vi "TIO Stream Read_Ser.vi"(8 "error in (no error)":errorcluster, 11 "VISA resource name":refnum<visa-resource-name>) -> (0 "error out":errorcluster, 1 "Payload":string, 2 "Type":T1(ring)=enum."RPC Request", 3 "VISA resource name Out":refnum<visa-resource-name>, 4 "Payload Length":u16)   [LabVIEW 2019]
uses:
  <userlib>/TIO Library 2010/TIO Serial Checksum CRC32.vi
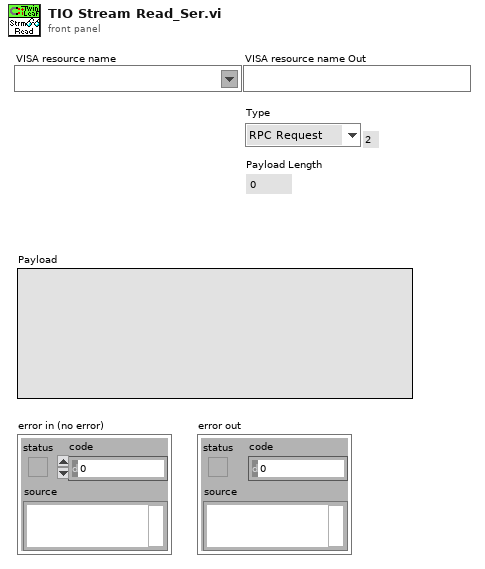
[diagram p1: front panel]
types:
  T1 = enum8{"Invalid", "Log", "RPC Request", "RPC Reply", "RPC Error", "Stream Description", "User"}
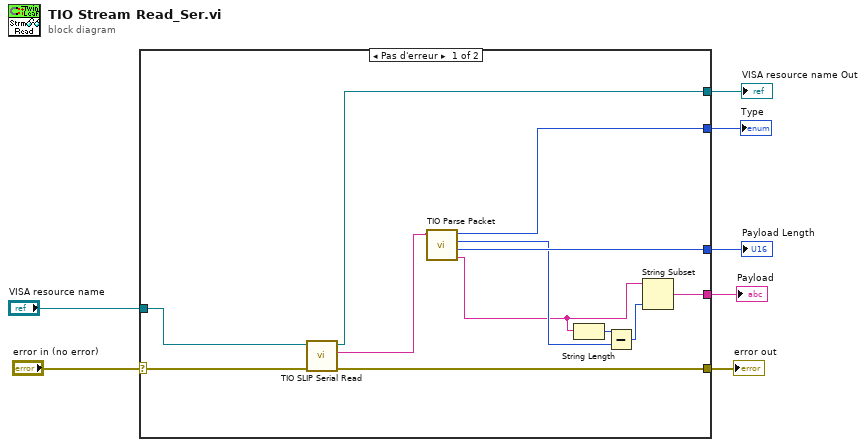
[diagram p0: block diagram]
diagram:
  n1 = case shown="Pas d'erreur" "error in (no error)" {
    selector: "error in (no error)" -> [w9 w20]
    tunnel: [w19 w20] -> w7
    tunnel: [w18 _] -> w6
    tunnel: [w17 _] -> w5
    tunnel: [w12 _] -> w4
    tunnel: "VISA resource name" -> [w10 w21]
    tunnel: [w8 w21] -> w1
    frame No Error {
      n2 = call <userlib>:"TIO SLIP Serial Read.vi"("error in (no error)"=w9, "VISA resource name"=w10) -> ("error out"=w19:errorcluster, "Payload"=w11:string, "VISA resource name Out"=w8:refnum<visa-resource-name>)  [unwired: 6 in, 1 out]
      n3 = call <userlib>:"TIO Parse Packet.vi"("Packet"=w11) -> ("Payload"=w13:string, "Payload Length"=w18:u16, "Routing Size"=w14:u8, "Type"=w17:u16)  [unwired: 7 in]
      n4 = String Length(string=w13) -> (length=w16:i32)
      n5 = Subtract(x=w16, y=w14) -> (x-y=w15:i32)
      n6 = String Subset(string=w13, length (rest)=w15) -> (substring=w12:string)  [unwired: 1 in]
    }
    frame Error {
    }
  }
  "error out" <- w7
  "Payload" <- w4
  "Type" <- w5
  "Payload Length" <- w6
  "VISA resource name Out" <- w1
